vi "UHR-Fleezers Control (host) - 12.0_test_fpga_connection.vi"() -> ()   [LabVIEW 2014] (continued)
                    frame 3 {
                      n2355 = local read "Trap D (MHz)"() -> (w3391:dbl)
                      n2356 = property on="Initial D (MHz)" class="DigNum (strict)"("Val(Sgnl)"=w3391) -> ()  [unwired: 2 in, 2 out]
                      n2357 = local write "Manipulating Trap"(FALSE ("Manipulating Trap")) -> ()
                    }
                  }
                }
              }
            }
          }
        }
      }
      event Mouse Move {
        n2358 = event-data() -> ()  [unwired: 6 out]
      }
    }
    n2359 = local read "Stop All"() -> (w3174:bool)
    n2360 = node-c288() -> ()  [unwired: 2 out]
  }
  n2361 = node-c288(w136) -> ()  [unwired: 1 out]
  n2362 = node-c288(w138) -> ()  [unwired: 1 out]
  n2363 = node-c288(w125) -> ()  [unwired: 1 out]
  n2364 = flat-sequence "Video" {
    tunnel: [w3402] -> w127
    tunnel: w127 -> [w3443]
    frame #0 {
      n2365 = while {
        stop <- w3395 continue-if-true
        n2366 = call "Close Video Capture.vi"() -> ("error code OUT"=w3397:i32)
        n2367 = Equal?(x=w3397, y=0) -> (x = y?=w3395:bool)
      }
      n2368 = local write "Stop All"(FALSE ("Stop All")) -> ()
    }
    frame #1 {
      n2369 = call "DMR_Init.vi"() -> ()  [unwired: 3 out]
    }
    frame #2 {
      # "Setting the destination format to Mono8 makes sure that the image can be displayed in the intensity plot."
      n2370 = call "DMR_GetDevice.vi"("search string IN"="DE019116701") -> ("device handle OUT"=w3420:i32)  [unwired: 4 in, 2 out]
      n2371 = call "DMR_OpenDevice.vi"("device handle IN"=w3420) -> ("driver handle OUT"=w3403:i32)  [unwired: 4 out]
      n2372 = call "DMR_FindList.vi"("flags IN"=u32 0 ("flags"), "list name IN"="" ("String"), "list type IN"=T38."camera descriptions", "driver handle IN"=w3403) -> ("list handle OUT"=w3406:i32)  [unwired: 2 out]
      n2373 = call "DMR_FindList.vi"("flags IN"=u32 0 ("flags"), "list name IN"="Base", "list type IN"=T38."setting", "driver handle IN"=w3403) -> ("list handle OUT"=w3404:i32)  [unwired: 2 out]
      n2374 = call "OBJ_GetHandle.vi"("object name IN"="VideoStandard", "list handle IN"=w3406) -> ("object handle OUT"=w3400:i32)  [unwired: 3 out]
      n2375 = call "OBJ_GetHandle.vi"("object name IN"="PixelFormat", "list handle IN"=w3404) -> ("object handle OUT"=w3414:i32)  [unwired: 3 out]
      n2376 = call "OBJ_SetS.vi"("value index IN"=0, "value IN"="NTSC M", "object handle IN"=w3400) -> ()  [unwired: 2 out]
      n2377 = call "OBJ_SetS.vi"("value index IN"=0, "value IN"="Mono8" ("value"), "object handle IN"=w3414) -> ()  [unwired: 2 out]
      n2378 = call "OBJ_GetHandle.vi"("object name IN"="VideoChannel", "list handle IN"=w3404) -> ("object handle OUT"=w3410:i32)  [unwired: 3 out]
      n2379 = while {
        tunnel: [w3425] -> w3402
        tunnel: w3403 -> [w3422]
        stop <- w3423 continue-if-true
        n2380 = call "DMR_ImageRequestSingle.vi"("request control IN"=0, "driver handle IN"=w3422) -> ("error code OUT"=w3424:i32, "driver handle OUT"=w3425:i32)  [unwired: 2 out]
        n2381 = Equal To 0?(x=w3424) -> (x = 0?=w3423:bool)
      }
      n2382 = call "OBJ_SetI.vi"("value index IN"=0, "value IN"=3 ("Video channel"), "object handle IN"=w3410) -> ()  [unwired: 2 out]
    }
    frame #3 {
      w3431 = T20 0 items=["Grayscale (U8)", "Grayscale (I16)", "Grayscale (SGL)", "Complex (CSG)", "RGB (U32)", "HSL (U32)", "RGB (U64)"] ("Image Type")
      w3439 = T20 0 items=["Grayscale (U8)", "Grayscale (I16)", "Grayscale (SGL)", "Complex (CSG)", "RGB (U32)", "HSL (U32)", "RGB (U64)"] ("Image Type")
      n2383 = for "Create Greyscale map" {
        N: 256 -> [_]
        tunnel: [w3445] -> w3428 mode=indexing
        workers-P: _ -> [_]
        i -> [w3448]
        n2384 = To Unsigned Byte Integer(number=w3448) -> (unsigned 8bit integer=w3444:u8)
        n2385 = Join Numbers(hi=w3444, lo=w3444) -> ((hi.lo)=w3447:u16)
        n2386 = Join Numbers(hi=w3444, lo=w3444) -> ((hi.lo)=w3446:u16)
        n2387 = Join Numbers(hi=w3447, lo=w3446) -> ((hi.lo)=w3445:u32)
      }
      n2388 = call "IMAQ Create"("Image Name"="Scaled video", "Image Type"=w3431) -> ("New Image"=w3430:T2)  [unwired: 2 in, 2 out]
      n2389 = call "IMAQ Create"("Image Name"="Main video", "Image Type"=w3439) -> ("New Image"=w3440:T2)  [unwired: 2 in, 2 out]
      n2390 = node-c288(0 ("Processor")) -> (w3438:T26)  [unwired: 3 out]
      n2391 = Initialize Array(u32 0 ("Window Number (0...15)"), 480 ("dimension size"), 640 ("dimension size")) -> (w3433:u32[][])
      n2392 = timed-loop {
        tunnel: w3443 -> [w3465]
        tunnel: [w3464] -> w3442
        tunnel: w3440 -> [w3463]
        timing: w3438 -> [_]
        timing-out: [_] -> w3437
        tunnel: w3433 -> [w3452]
        tunnel: w3430 -> [w3450]
        tunnel: w3428 -> [w3449]
        stop <- w3451 stop-if-true
        # "This block performs the \nactual image capture."
        n2393 = node-c288() -> ()  [unwired: 2 out]
        n2394 = local read "Stop All"() -> (w3451:bool)
        n2395 = Reciprocal(x="Video Capture Rate (Hz)") -> (1/x=w3455:dbl)
        n2396 = Multiply(x=w3455, y=1000.0) -> (x*y=w3453:dbl)
        n2397 = call "DMR_ImageRequestWaitFor.vi"("queue number IN"=0, "timeout(ms) IN"=500, "driver handle IN"=w3465) -> ("error code OUT"=w3469:i32, "request number OUT"=w3466:i32, "driver handle OUT"=w3467:i32)
        n2398 = feedback #1(T39 refnum ("Avi Refnum")) -> (w3457:T39)
        n2399 = case shown="True" "New Video File" {
          tunnel: [T39 refnum ("Avi Refnum") w3486] -> w3459
          tunnel: [FALSE TRUE] -> w3460
          tunnel: w3457 -> [_ w3482]
          frame False {
          }
          frame True {
            n2400 = call "Create new save file.vi"("Ext"=".avi" ("string"), "Index In"="Video Index") -> ("Path Out"=w3478:path, "Index Out"=w3479:dbl)  [unwired: 1 in]
            "Path Out" <- w3478
            n2401 = Not Equal?(x=w3482, y=T39 refnum ("Avi Refnum")) -> (x != y?=w3483:bool)
            n2402 = Increment(x=w3479) -> (x+1=w3488:dbl)
            n2403 = case shown="True" w3483 {
              tunnel: w3482 -> [_ w3489]
              frame False {
              }
              frame True {
                n2404 = call "IMAQ AVI Close"("Avi Refnum"=w3489) -> ()  [unwired: 1 in, 10 out]
              }
            }
            n2405 = local write "Video Index"(w3488) -> ()
            n2406 = call "IMAQ AVI Create"("Frames Per Second"=u32 30, "AVI Path"=w3478) -> ("Avi Refnum"=w3486:T39)  [unwired: 5 in, 4 out]
          }
        }
        n2407 = Equal To 0?(x=w3469) -> (x = 0?=w3468:bool)
        n2408 = Select(t=w3459, s=w3460, f=w3457) -> (s? t:f=w3458:T39)
        n2409 = feedback-in #1(w3458) -> ()
        n2410 = case shown="True" w3468 {
          tunnel: w3467 -> [w3490 w3517]
          tunnel: w3466 -> [_ w3516]
          tunnel: [w3490 w3513] -> w3464
          tunnel: w3463 -> [_ w3494]
          tunnel: w3452 -> [_ w3501]
          tunnel: w3458 -> [_ w3499]
          tunnel: w3450 -> [_ w3495]
          tunnel: w3449 -> [_ w3496]
          frame False {
          }
          frame True {
            w3507 = u32 0 ("X-offset IN")
            n2411 = call "DMR_GetImageRequestBufferData.vi"("driver handle IN"=w3517, "request number IN"=w3516) -> ("width OUT"=w3506:i32, "height OUT"=w3505:i32, "driver handle OUT"=w3512:i32, "request number OUT"=w3511:i32, "bytes per pixel OUT"=w3508:i32)  [unwired: 13 out]
            n2412 = call "DMR_GetImageRequestBufferImageData.vi"("driver handle IN"=w3512, "request number IN"=w3511, "bytes per pixel IN"=w3508, "X-offset IN"=w3507, "Y-offset IN"=w3507, "height IN"=w3505, "width IN"=w3506) -> ("driver handle OUT"=w3510:u32, "request number OUT"=w3509:u32, "image OUT"=w3502:u32[][])  [unwired: 10 out]
            n2413 = call "DMR_ImageRequestUnlock.vi"("request number IN"=w3509, "driver handle IN"=w3510) -> ("driver handle OUT"=w3515:i32)  [unwired: 1 in, 2 out]
            n2414 = case shown="True" "Averaging" {
              tunnel: w3502 -> [w3558 w3563]
              tunnel: [w3558 w3562] -> w3498
              tunnel: w3501 -> [_ w3560]
              frame False {
              }
              frame True {
                (unwired) 1
                w3568 = 1
                n2415 = feedback #2(w3560) -> (w3559:u32[][])
                n2416 = Add(x=w3563, y=w3559) -> (x+y=w3564:u32[][])
                n2417 = Select(t=w3560, s="Reset Averaging", f=w3564) -> (s? t:f=w3566:u32[][])
                n2418 = feedback-in #2(w3566) -> ()
                n2419 = feedback #3(w3568) -> (w3561:i32)
                n2420 = Divide(x=w3564, y=w3561) -> (x/y=w3565:dbl[][])
                n2421 = Increment(x=w3561) -> (x+1=w3569:i32)
                n2422 = To Unsigned Long Integer(number=w3565) -> (unsigned 32bit integer=w3562:u32[][])
                n2423 = Select(t=w3568, s="Reset Averaging", f=w3569) -> (s? t:f=w3567:i32)
                n2424 = feedback-in #3(w3567) -> ()
              }
            }
            n2425 = call "DMR_ImageRequestSingle.vi"("request control IN"=0, "driver handle IN"=w3515) -> ("driver handle OUT"=w3513:i32)  [unwired: 3 out]
            n2426 = disable-structure shown="Disabled" {
              disable-tunnel: w3498 -> [w3535 _]
              disable-tunnel: w3495 -> [w3534 _]
              frame Disabled {
                n2427 = To Double Precision Float(number=w3535) -> (double precision float=w3533:dbl[][])
                n2428 = In Range and Coerce(upper limit="Intensity Upper", x=w3533, lower limit="Intensity Lower") -> (coerced(x)=w3532:dbl[][])  [unwired: 1 out]
                n2429 = Subtract(x="Intensity Upper", y="Intensity Lower") -> (x-y=w3529:dbl)
                n2430 = Subtract(x=w3532, y="Intensity Lower") -> (x-y=w3530:dbl[][])
                n2431 = Divide(x=w3530, y=w3529) -> (x/y=w3531:dbl[][])
                n2432 = Multiply(x=255.0, y=w3531) -> (x*y=w3527:dbl[][])
                n2433 = To Unsigned Byte Integer(number=w3527) -> (unsigned 8bit integer=w3536:u8[][])
                n2434 = call "IMAQ ArrayToImage"("Image Pixels (U8)"=w3536, "Image"=w3534) -> ("Image Out"=w3523:T2)  [unwired: 4 in, 5 out]
                n2435 = First Call?() -> (First Call?: T/F=w3524:bool)
                n2436 = case shown="True" w3524 {
                  tunnel: w3523 -> [w3537 w3548]
                  frame False {
                    n2437 = flat-sequence {
                      tunnel: w3537 -> [w3543]
                      frame #0 {
                        w3540 = FALSE ("Get/Set Status? (Set)")
                        w3539 = 0 ("Window Number (0...15)")
                        n2438 = call "IMAQ WindSize"("Get/Set Status? (Set)"=w3540, "Window Number"=w3539) -> ("Width & Height out"=→"Window Size":cluster{"Width":i32, "Height":i32})  [unwired: 4 in, 2 out]
                        n2439 = call "IMAQ WindMove"("Window Number (0...15)"=w3539, "Get/Set Status? (Set)"=w3540) -> ("Coordinates (screen)"=→"Window Position":cluster{"X Position":i32, "Y Position":i32})  [unwired: 3 in, 1 out]
                        n2440 = call "IMAQ WindDraw"("Resize to Image Size? (Y)"=FALSE, "Window Number (0...15)"=w3539, "Image"=w3543) -> ()  [unwired: 7 in, 2 out]
                      }
                      frame #1 {
                        n2441 = call "IMAQ WindZoom 2"("Center Point"="Center Point", "Zoom to Fit? (False)"=FALSE, "Zoom Factor"="Zoom Factor") -> ()  [unwired: 5 in, 4 out]
                      }
                    }
                  }
                  frame True {
                    n2442 = flat-sequence {
                      tunnel: w3548 -> [w3551]
                      tunnel: [w3549] -> w3547
                      tunnel: w3547 -> [w3553]
                      frame #0 {
                        w3550 = TRUE ("Resize to Image Size? (Y)")
                        w3549 = 0 ("Window Number (0...15)")
                        n2443 = call "IMAQ WindNonTearing"("Window Number"=w3549, "NonTearing? (True)"=w3550) -> ()  [unwired: 8 in, 2 out]
                        n2444 = call "IMAQ WindDraw"("Resize to Image Size? (Y)"=w3550, "Window Number (0...15)"=w3549, "Image"=w3551) -> ()  [unwired: 7 in, 2 out]
                      }
                      frame #1 {
                        n2445 = call "IMAQ WindSize"("Scrollbars? (N)"=FALSE, "Width & Height"="Initial Window Size", "Window Number"=w3553) -> ()  [unwired: 3 in, 3 out]
                        n2446 = call "IMAQ WindMove"("Window Number (0...15)"=w3553, "Coordinates (screen)"="Initial Window Position") -> ()  [unwired: 3 in, 2 out]
                      }
                    }
                  }
                }
              }
              frame Enabled {
              }
            }
            n2447 = To Unsigned Byte Integer(number=w3498) -> (unsigned 8bit integer=w3497:u8[][])
            n2448 = call "IMAQ ArrayToImage"("Image Pixels (U8)"=w3497, "Image"=w3494) -> ("Image Out"=w3492:T2)  [unwired: 4 in, 5 out]
            n2449 = case shown="True" "Save Video" {
              tunnel: w3499 -> [_ w3557]
              tunnel: w3492 -> [_ w3556]
              frame False {
              }
              frame True {
                n2450 = call "IMAQ AVI Write Frame"("Image"=w3556, "Avi Refnum"=w3557) -> ()  [unwired: 2 in, 8 out]
              }
            }
            n2451 = case shown="True" "Save Image" {
              tunnel: w3497 -> [_ w3572]
              tunnel: w3496 -> [_ w3571]
              frame False {
              }
              frame True {
                n2452 = call <vilib>:"Flatten Pixmap.vi"("colors"=w3571, "8-bit pixmap"=w3572) -> ("image data"=w3578:T40)  [unwired: 4 in, 5 out]
                n2453 = call "Create new save file.vi"("Insert"="video_frame_" ("string"), "Ext"=".bmp" ("string"), "Index In"="Image Index") -> ("Path Out"=w3574:path, "Index Out"=w3579:dbl)
                n2454 = Increment(x=w3579) -> (x+1=w3573:dbl)
                n2455 = local write "Image Index"(w3573) -> ()
                n2456 = call <vilib>:"Write BMP File.vi"("image data"=w3578, "path to BMP file"=w3574) -> ()  [unwired: 1 in, 9 out]
              }
            }
            n2457 = case shown="True" "Target" {
              tunnel: w3492 -> [w3518 w3522]
              tunnel: [w3518 w3520] -> w3491
              frame False {
              }
              frame True {
                n2458 = local read "Target coordinates"() -> (w3519:cluster{"X1":dbl, "Y1":dbl, "X2":dbl, "Y2":dbl})
                n2459 = call "IMAQ Overlay Oval"("Color"=u32 16711680, "Bounding Rectangle"=w3519, "Image"=w3522) -> ("Image Out"=w3520:T2)  [unwired: 7 in, 1 out]
              }
            }
            "Primary Video Display" <- w3491
          }
        }
        n2460 = node-c288(w3453) -> ()  [unwired: 1 out]
      }
      n2461 = node-c288(w3437) -> ()  [unwired: 1 out]
      n2462 = call "DMR_CloseDevice2.vi"("driver handle IN"=w3442) -> ()  [unwired: 1 in, 4 out]
    }
    frame #4 {
      n2463 = call "DMR_Close.vi"() -> ()  [unwired: 1 out]
    }
  }
  n2464 = local write "Offset (nm)"(0.0 ("Offset (nm)")) -> ()
  n2465 = local write "Bead Mean (nm)"(0.0 ("Bead Mean (nm)")) -> ()
  n2466 = local write "Total Volume\nFlowed P1 (uL)"(w45) -> ()
  n2467 = local write "Total Volume\nFlowed Samp (uL)"(w45) -> ()
  n2468 = local write "Total Volume\nFlowed P3 (uL)"(w45) -> ()
  n2469 = node-c288(i64 1 ("Period"), 1 ("Processor")) -> (w217:T26)  [unwired: 2 out]
  n2470 = timed-loop "Acquire Data" {
    tunnel: w51 -> [w3886]
    tunnel: w98 -> [w3885]
    tunnel: [w3915] -> w309
    tunnel: [w3910] -> w307
    timing: w217 -> [_]
    timing-out: [_] -> w216
    tunnel: w116 -> [w3742]
    stop <- "Stop All" stop-if-true
    w3666 = "Initialize"
    w3732 = "NI_ChannelName" ("name")
    # "I think that the conversion\nfrom 'wiggle amp' to nm\nis 0.277 nm/input. So, 1000\nfor an input is 277 nm."
    n2471 = node-c288() -> ()  [unwired: 2 out]
    n2472 = First Call?() -> (First Call?: T/F=w3701:bool)
    n2473 = Or(x="Reset", y=w3701) -> (x .or. y?=w3702:bool)
    n2474 = local read "Flushing P1"() -> (w3621:bool)
    n2475 = case "Reset data stream" shown="True" w3702 {
      tunnel: w3886 -> [w4951 w4959]
      tunnel: w3885 -> [w4950 w4958]
      tunnel: [w4951 w4953] -> w3614
      tunnel: [w4950 w4952] -> w3881
      frame False {
      }
      frame True {
        w4956 = TRUE ("AI to FIFO")
        n2476 = local write "Overflow (data lost)"(FALSE ("Overflow (data lost)")) -> ()
        n2477 = call "reset FPGA DMA.vi"("error in"=w4958, "FPGA VI Reference In"=w4959) -> ("error out"=w4954:errorcluster, "FPGA VI Reference Out"=w4955:T22)
        n2478 = xnode "Read/Write Control"("FPGA VI Reference In"=w4955, "error in"=w4954, "AI to FIFO"=w4956, "APD to FIFO"=w4956) -> ("FPGA VI Reference Out"=w4953:T22, "error out"=w4952:errorcluster)
      }
    }
    n2479 = case shown="True" w3621 {
      frame False {
      }
      frame True {
        n2480 = local read "Flush rate (uL/m) P1"() -> (w3986:dbl)
        n2481 = local read "HP1 Flush Time (s)"() -> (w3992:dbl)
        n2482 = local read "DMA Update Period (s)"() -> (w3979:dbl)
        n2483 = Divide(x=w3986, y=60.0) -> (x/y=w3978:dbl)
        n2484 = feedback #4(0.0) -> (w3981:dbl)
        n2485 = Divide(x=w3992, y=w3979) -> (x/y=w3984:dbl)
        n2486 = feedback #5(0) -> (w3990:i32)
        n2487 = Increment(x=w3990) -> (x+1=w3983:i32)
        n2488 = Multiply(x=w3979, y=w3978) -> (x*y=w3977:dbl)
        n2489 = Greater?(x=w3983, y=w3984) -> (0:w3989:bool)
        n2490 = Compound Arithmetic op=MULTIPLY(w3979, w3983, w3978) -> (→"P1 Flush Volume (uL)":dbl)
        n2491 = Divide(x=w3983, y=w3984) -> (x/y=→"P1 Flushing Bar":dbl)
        n2492 = Add(x=w3977, y=w3981) -> (x+y=w3980:dbl)
        "Total Volume\nFlowed P1 (uL)" <- w3980
        n2493 = feedback-in #4(w3980) -> ()
        n2494 = case shown="True" w3989 {
          tunnel: w3983 -> [w3993 _]
          tunnel: [w3993 0] -> w3988
          frame False {
          }
          frame True {
            w3994 = FALSE ("Flushing P1")
            n2495 = local write "Inject Pump 1"(w3994) -> ()
            n2496 = local write "Flushing P1"(w3994) -> ()
            n2497 = property on="Clear Volume P1" class="Bool (strict)"("Val(Sgnl)"=TRUE ("Value (Signaling)")) -> ()  [unwired: 2 in, 2 out]
          }
        }
        n2498 = feedback-in #5(w3988) -> ()
      }
    }
    n2499 = Or(x="Start AOD Scan", y="Trap Raster Scan") -> (x .or. y?=w3840:bool)
    n2500 = case "Start AOM raster scan" shown="True" w3840 {
      tunnel: w3614 -> [w4801 w4811]
      tunnel: w3881 -> [w4800 w4810]
      tunnel: [w4801 w4804] -> w3606
      tunnel: [w4800 w4803] -> w3880
      frame False {
      }
      frame True {
        n2501 = case shown="True" "Restart DMA? (AOD)" {
          tunnel: [w4849 w4851] -> w4805
          tunnel: [w4848 w4850] -> w4806
          tunnel: w4811 -> [w4849 w4853]
          tunnel: w4810 -> [w4848 w4852]
          frame False {
          }
          frame True {
            n2502 = local write "Overflow (data lost)"(FALSE ("Overflow (data lost)")) -> ()
            n2503 = call "reset FPGA DMA.vi"("error in"=w4852, "FPGA VI Reference In"=w4853) -> ("error out"=w4850:errorcluster, "FPGA VI Reference Out"=w4851:T22)
          }
        }
        n2504 = local write "Trap Raster Scan"(FALSE ("Trap Raster Scan")) -> ()
        n2505 = case shown="False" "Move MCL Also?" {
          tunnel: w4806 -> [w4815 w4843]
          tunnel: w4805 -> [w4816 w4844]
          tunnel: [w4814 w4847] -> w4804
          tunnel: [w4813 w4846] -> w4803
          frame False {
            w4812 = TRUE ("AI to FIFO")
            n2506 = xnode "Read/Write Control"("FPGA VI Reference In"=w4816, "error in"=w4815, "AI to FIFO"=w4812, "APD to FIFO"=w4812, "Start scan"=w4812) -> ("FPGA VI Reference Out"=w4814:T22, "error out"=w4813:errorcluster)
          }
          frame True {
            w4840 = FALSE ("1D or 2D Scan?")
            w4845 = TRUE ("AI to FIFO")
            # "Count for MCL loop"
            # "N total cycles"
            # "N steps"
            # "V_int"
            n2507 = local read "Scan Range (nm)"() -> (w4822:dbl)
            n2508 = local read "Number of F/B Scans (AOD)"() -> (w4839:u16)
            n2509 = Sign(1:w4822) -> (0:w4821:dbl)
            n2510 = Compound Arithmetic op=MULTIPLY(w4822, "MCL Step Position Ratio", "MCL/AOM Scale Tweak") -> (w4826:dbl)
            n2511 = Negate(x=w4821) -> (-x=w4818:dbl)
            n2512 = Multiply(x=w4818, y="MCL Step Increment (V_int)") -> (x*y=w4820:dbl)
            n2513 = Divide(x=w4826, y="MCL X Cal (nm/V)") -> (x/y=w4832:dbl)
            n2514 = Multiply(x=32767.0 ("y"), y=w4832) -> (x*y=w4838:dbl)
            n2515 = local read "Total Counts (ticks)"() -> (w4823:u32)
            n2516 = local read "Cycles/step (AOD)"() -> (w4834:u64)
            n2517 = local read "Scan steps (AOD)"() -> (w4835:u64)
            n2518 = Divide(x=w4838, y=10.0) -> (x/y=w4831:dbl)
            n2519 = Divide(x=w4831, y="MCL Step Increment (V_int)") -> (x/y=w4829:dbl)
            n2520 = Absolute Value(x=w4829) -> (abs(x)=w4817:dbl)
            n2521 = Compound Arithmetic op=MULTIPLY(w4835, w4834, w4823) -> (w4830:u64)
            n2522 = local write "wait to reset values"(w4845) -> ()
            n2523 = local write "MCL Scanning"(w4845) -> ()
            n2524 = Divide(x=w4830, y=w4817) -> (x/y=w4827:dbl)
            "MCL Count" <- w4827
            n2525 = xnode "Read/Write Control"("FPGA VI Reference In"=w4844, "error in"=w4843, "Scan steps (MCL)"=w4817, "Number of scans (MCL)"=w4839, "Cycles per step (MCL)"=u64 1, "Scan freq.  increment (MCL)"=w4820, "1D or 2D Scan?"=w4840, "MCL Scan Axis"=w4840, "Cont. Scan (MCL)"=w4840, "MCL count"=w4827) -> ("FPGA VI Reference Out"=w4842:T22, "error out"=w4841:errorcluster)
            n2526 = xnode "Read/Write Control"("FPGA VI Reference In"=w4842, "error in"=w4841, "AI to FIFO"=w4845, "APD to FIFO"=w4845, "Start scan"=w4845, "Start scan (MCL)"=w4845) -> ("FPGA VI Reference Out"=w4847:T22, "error out"=w4846:errorcluster)
          }
        }
        "Raster Scanning..." <- TRUE ("Scanning...")
      }
    }
    n2527 = local read "Flushing P3"() -> (w3622:bool)
    n2528 = case "Keep track of when Harvard Pump 3 is done flushing" shown="True" w3622 {
      frame False {
      }
      frame True {
        n2529 = local read "Flush rate (uL/m) P3"() -> (w4005:dbl)
        n2530 = local read "DMA Update Period (s)"() -> (w3999:dbl)
        n2531 = local read "HP3 Flush Time (s)"() -> (w4013:dbl)
        n2532 = Divide(x=w4005, y=60.0) -> (x/y=w4000:dbl)
        n2533 = feedback #6(0) -> (w4011:i32)
        n2534 = Increment(x=w4011) -> (x+1=w4006:i32)
        n2535 = Divide(x=w4013, y=w3999) -> (x/y=w4007:dbl)
        n2536 = Multiply(x=w3999, y=w4000) -> (x*y=w3998:dbl)
        n2537 = Greater?(x=w4006, y=w4007) -> (0:w4010:bool)
        n2538 = feedback #7(0.0) -> (w4001:dbl)
        n2539 = Compound Arithmetic op=MULTIPLY(w3999, w4006, w4000) -> (→"P3 Flush Volume (uL)":dbl)
        n2540 = case shown="True" w4010 {
          tunnel: w4006 -> [w4014 _]
          tunnel: [w4014 0] -> w4009
          frame False {
          }
          frame True {
            w4015 = FALSE ("Flushing P3")
            n2541 = local write "Inject Pump 3"(w4015) -> ()
            n2542 = local write "Flushing P3"(w4015) -> ()
            n2543 = property on="Clear Volume P3" class="Bool (strict)"("Val(Sgnl)"=TRUE ("Value (Signaling)")) -> ()  [unwired: 2 in, 2 out]
          }
        }
        n2544 = feedback-in #6(w4009) -> ()
        n2545 = Divide(x=w4006, y=w4007) -> (x/y=→"P3 Flushing Bar":dbl)
        n2546 = Add(x=w3998, y=w4001) -> (x+y=w4002:dbl)
        "Total Volume\nFlowed P3 (uL)" <- w4002
        n2547 = feedback-in #7(w4002) -> ()
      }
    }
    n2548 = And(x="Save scans", y=w3840) -> (x .and. y?=w3879:bool)
    n2549 = local read "Flushing samp"() -> (w3615:bool)
    n2550 = case shown="True" w3615 {
      frame False {
      }
      frame True {
        n2551 = local read "DMA Update Period (s)"() -> (w3958:dbl)
        n2552 = local read "Flush rate (mL/m)"() -> (w3970:dbl)
        n2553 = local read "Samp Flush Time (s)"() -> (w3971:dbl)
        n2554 = Divide(x=w3970, y=60.0) -> (x/y=w3957:dbl)
        n2555 = feedback #8(0) -> (w3963:i32)
        n2556 = Increment(x=w3963) -> (x+1=w3962:i32)
        n2557 = Divide(x=w3971, y=w3958) -> (x/y=w3967:dbl)
        n2558 = Multiply(x=w3958, y=w3957) -> (x*y=w3956:dbl)
        n2559 = Greater?(x=w3962, y=w3967) -> (0:w3966:bool)
        n2560 = feedback #9(0.0) -> (w3959:dbl)
        n2561 = Compound Arithmetic op=MULTIPLY(w3958, w3962, w3957) -> (→"Samp Volume (uL)":dbl)
        n2562 = Divide(x=w3962, y=w3967) -> (x/y=→"Samp flush bar":dbl)
        n2563 = case shown="True" w3966 {
          tunnel: [w3972 0] -> w3965
          tunnel: w3962 -> [w3972 _]
          frame False {
          }
          frame True {
            w3975 = FALSE ("Flushing samp")
            n2564 = local write "Sample Channel\nFlow"(w3975) -> ()
            n2565 = local write "Flushing samp"(w3975) -> ()
            n2566 = property on="Clear Volume" class="Bool (strict)"("Val(Sgnl)"=TRUE) -> ()  [unwired: 2 in, 2 out]
          }
        }
        n2567 = feedback-in #8(w3965) -> ()
        n2568 = Add(x=w3956, y=w3959) -> (x+y=w3960:dbl)
        "Total Volume\nFlowed Samp (uL)" <- w3960
        n2569 = feedback-in #9(w3960) -> ()
      }
    }
    n2570 = Compound Arithmetic op=OR("Start MCL Scan", "Confocal\nImage", "Confocal\nLinescan") -> (w3838:bool)
    n2571 = And(x="Save Data (MCL)", y=w3838) -> (x .and. y?=w3878:bool)
    n2572 = case "Start MCL raster scan" shown="True" w3838 {
      tunnel: w3606 -> [w4420 w4436]
      tunnel: w3880 -> [w4419 w4435]
      tunnel: [w4420 w4431] -> w3613
      tunnel: [w4419 w4430] -> w3611
      tunnel: [FALSE w4429] -> w3864
      tunnel: "Start MCL Scan" -> [_ w4424]
      tunnel: "Confocal\nImage" -> [_ w4423]
      tunnel: "Confocal\nLinescan" -> [_ _]
      frame False {
      }
      frame True {
        w4429 = TRUE
        n2573 = case shown="True" "Restart DMA? (MCL)" {
          tunnel: [w4481 w4483] -> w4434
          tunnel: [w4480 w4482] -> w4433
          tunnel: w4436 -> [w4481 w4486]
          tunnel: w4435 -> [w4480 w4485]
          frame False {
          }
          frame True {
            n2574 = call "reset FPGA DMA.vi"("error in"=w4485, "FPGA VI Reference In"=w4486) -> ("error out"=w4482:errorcluster, "FPGA VI Reference Out"=w4483:T22)
            n2575 = local write "Overflow (data lost)"(FALSE ("Overflow (data lost)")) -> ()
          }
        }
        n2576 = case shown="False" w4424 {
          selector: w4424 -> [_ w4440]
          tunnel: w4423 -> [w4439 _]
          tunnel: [w4439 w4440] -> w4422
          frame False {
            n2577 = property on="2D or 1D Scan" class="Bool (strict)"("Val(Sgnl)"=w4439) -> ()  [unwired: 2 in, 2 out]
            n2578 = property on="Confocal\nImage" class="Bool (strict)"("Value"=FALSE ("Start Confocal Map")) -> ()  [unwired: 2 in, 2 out]
          }
          frame True {
          }
        }
        n2579 = local write "MCL Scanning"(w4429) -> ()
        n2580 = local read "AO1"() -> (w4426:dbl)
        n2581 = local read "AO2"() -> (w4425:dbl)
        n2582 = case shown="True" "Center Scan" {
          tunnel: w4434 -> [w4447 w4479]
          tunnel: w4433 -> [w4446 w4478]
          tunnel: [w4445 w4477] -> w4431
          tunnel: [w4444 w4476] -> w4430
          tunnel: [w4442 w4463] -> w4428
          tunnel: [w4441 w4462] -> w4427
          tunnel: w4426 -> [w4442 w4468]
          tunnel: w4425 -> [w4441 w4471]
          tunnel: w4422 -> [_ _]
          frame False {
            w4443 = TRUE ("AI to FIFO")
            n2583 = xnode "Read/Write Control"("FPGA VI Reference In"=w4447, "error in"=w4446, "AI to FIFO"=w4443, "APD to FIFO"=w4443, "Start scan (MCL)"=w4443) -> ("FPGA VI Reference Out"=w4445:T22, "error out"=w4444:errorcluster)
          }
          frame True {
            w4475 = TRUE ("AI to FIFO")
            n2584 = local read "Scan steps (MCL)"() -> (w4454:u64)
            n2585 = local read "Scan lines (y)"() -> (w4450:u64)
            n2586 = local read "Fast Scan Dir"() -> (w4461:bool)
            n2587 = local read "Actual MCL Inc (V)"() -> (w4451:dbl)
            n2588 = Decrement(x=w4450) -> (x-1=w4449:u64)
            n2589 = Decrement(x=w4454) -> (x-1=w4453:u64)
            n2590 = Multiply(x=w4451, y=w4449) -> (x*y=w4448:dbl)
            n2591 = Divide(x=w4448, y=2.0) -> (x/y=w4458:dbl)
            n2592 = Multiply(x=w4451, y=w4453) -> (x*y=w4452:dbl)
            n2593 = Divide(x=w4452, y=2.0) -> (x/y=w4457:dbl)
            n2594 = Select(t=w4457, s=w4461, f=w4458) -> (s? t:f=w4456:dbl)
            n2595 = Select(t=w4458, s=w4461, f=w4457) -> (s? t:f=w4460:dbl)
            n2596 = Subtract(x=w4468, y=w4460) -> (x-y=w4459:dbl)
            n2597 = Subtract(x=w4471, y=w4456) -> (x-y=w4455:dbl)
            n2598 = local read "2D or 1D Scan"() -> (w4473:bool)
            n2599 = Not(x=w4461) -> (.not. x?=w4467:bool)
            n2600 = Not(x=w4473) -> (.not. x?=w4469:bool)
            n2601 = And(x=w4461, y=w4469) -> (x .and. y?=w4470:bool)
            n2602 = And(x=w4469, y=w4467) -> (x .and. y?=w4472:bool)
            n2603 = Select(t=w4471, s=w4472, f=w4455) -> (s? t:f=w4462:dbl)
            n2604 = Select(t=w4468, s=w4470, f=w4459) -> (s? t:f=w4463:dbl)
            n2605 = call "Volt to I16.vi"("Voltage In"=w4463) -> ("I16 Voltage Out"=w4466:i16)
            n2606 = call "Volt to I16.vi"("Voltage In"=w4462) -> ("I16 Voltage Out"=w4465:i16)
            n2607 = xnode "Read/Write Control"("FPGA VI Reference In"=w4479, "error in"=w4478, "AI to FIFO"=w4475, "APD to FIFO"=w4475, "Start scan (MCL)"=w4475, "AO1"=w4466, "AO2"=w4465) -> ("FPGA VI Reference Out"=w4477:T22, "error out"=w4476:errorcluster)
          }
        }
        "Initial Y" <- w4428
        "Initial X" <- w4427
        n2608 = local write "Tab Control 6"(T3."Imaging" ("Tab Control 6")) -> ()
        "wait to reset values" <- w4429
      }
    }
    n2609 = case shown="True" "Wiggle" {
      selector: "Wiggle" -> [w3929 _]
      tunnel: w3613 -> [w3931 w3944]
      tunnel: [w3928 w3947] -> w3612
      tunnel: w3611 -> [w3930 w3942]
      tunnel: [w3927 w3946] -> w3610
      frame False {
        n2610 = xnode "Read/Write Control"("FPGA VI Reference In"=w3931, "error in"=w3930, "Wiggle trap 1"=w3929) -> ("FPGA VI Reference Out"=w3928:T22, "error out"=w3927:errorcluster)
      }
      frame True {
        w3936 = FALSE ("Abort wiggle")
        w3940 = TRUE
        n2611 = local read "Restart DMA? (AOD)"() -> (w3945:bool)
        n2612 = case shown="True" w3945 {
          tunnel: w3944 -> [w3949 w3954]
          tunnel: [w3949 w3953] -> w3943
          tunnel: w3942 -> [w3948 w3952]
          tunnel: [w3948 w3951] -> w3941
          frame False {
          }
          frame True {
            n2613 = local write "Overflow (data lost)"(FALSE) -> ()
            n2614 = call "reset FPGA DMA.vi"("error in"=w3952, "FPGA VI Reference In"=w3954) -> ("error out"=w3951:errorcluster, "FPGA VI Reference Out"=w3953:T22)
          }
        }
        n2615 = local write "Wiggle"(FALSE) -> ()
        n2616 = xnode "Read/Write Control"("FPGA VI Reference In"=w3943, "error in"=w3941, "AI to FIFO"=w3940, "APD to FIFO"=w3940, "Wiggle trap 1"="Wiggle T1", "Wiggle freq 1 (Hz)"="Wiggle freq 1 (Hz)", "Wiggle amp 1"="Wiggle amp 1 (units?)", "Abort wiggle 1"=w3936, "Wiggle trap 2"="Wiggle T2", "Abort wiggle 2"=w3936, "Wiggle freq 2 (Hz)"="Wig Freq 2 (Hz)", "Wiggle amp 2"="Wig amp 2") -> ("FPGA VI Reference Out"=w3947:T22, "error out"=w3946:errorcluster)
      }
    }
    n2617 = local read "Trap Pos Elements/DMA read"() -> (w3596:u32)
    n2618 = local read "Trap AI Elements/DMA read"() -> (w3590:u32)
    n2619 = local read "APD Elements/DMA read"() -> (w3598:u32)
    n2620 = xnode "Get APD Data"("FPGA VI Reference In"=w3612, "error in"=w3610, "Number of Elements"=w3598, "Timeout (ms)"=-1) -> ("Data"=w3774:u32[], "Elements Remaining"=→"APD FIFO Elements Remaining":u32)  [unwired: 2 out]
    n2621 = xnode "Invoke Method"("FPGA VI Reference In"=w3612, "error in"=w3610, "Number of Elements"=w3596, "Timeout (ms)"=-1) -> ("Data"=w3705:u16[], "Elements Remaining"=→"Trap Pos FIFO El Remaining":u32)  [unwired: 2 out]
    n2622 = xnode "Get Trap Data"("FPGA VI Reference In"=w3612, "error in"=w3610, "Number of Elements"=w3590, "Timeout (ms)"=-1 ("Timeout")) -> ("FPGA VI Reference Out"=w3643:T22, "error out"=w3642:errorcluster, "Data"=w3706:i16[], "Elements Remaining"=w3589:u32)
    "FIFO El. Rem." <- w3589
    n2623 = local read "Trap AI FIFO Depth"() -> (w3924:u32)
    n2624 = Subtract(x=w3924, y=w3590) -> (x-y=w3923:u32)
    n2625 = Decimate 1D Array(w3705) -> (w3594:u16[], w3592:u16[], w3593:u16[])
    n2626 = Divide(x=w3589, y=w3923) -> (x/y=w3922:dbl)
    "Buffer Status" <- w3922
    n2627 = To Unsigned Long Integer(number=w3594) -> (unsigned 32bit integer=w3704:u32[])
    n2628 = Join Numbers(hi=w3592, lo=w3593) -> ((hi.lo)=w3703:u32[])
    n2629 = Equal?(x=w3922, y=1.0) -> (x = y?=w3920:bool)
    n2630 = Join Numbers(hi=w3704, lo=w3703) -> ((hi.lo)=w3697:u64[])
    n2631 = call "IR AOM word to freq - vec.vi"("Frequency Word In (double vec)"=w3697) -> ("Frequency Out"=w3740:dbl[])
    n2632 = case "Alert buffer overflow" shown="True" w3920 {
      frame False {
      }
      frame True {
        n2633 = call <vilib>:"Beep.vi"() -> ()  [unwired: 3 in, 9 out]
        "Overflow (data lost)" <- TRUE ("Overflow (data lost)")
      }
    }
    n2634 = Decimate 1D Array(w3740) -> (w3739:dbl[], w3738:dbl[])
    n2635 = Build Array(w3739, w3738) -> (w3737:dbl[][])
    n2636 = local read "Trap Sets"() -> (w3804:u32)
    n2637 = case "Deinterlace trap data, average down PSD" shown="2" w3804 {
      tunnel: w3706 -> [w4512 w4581]
      tunnel: [w4515 w4578] -> w3797
      tunnel: [w4512 w4580] -> w3700
      tunnel: "Detector Type" -> [w4517 w4576]
      tunnel: [w4516 w4579] -> w3796
      tunnel: [w4514 w4577] -> w3897
      frame 1, Default {
        n2638 = Divide(x=w4512, y=3276.7) -> (x/y=w4513:dbl[])
        n2639 = Decimate 1D Array(w4513) -> (w4526:dbl[], w4525:dbl[], w4524:dbl[], w4523:dbl[], w4522:dbl[], w4521:dbl[], w4520:dbl[], w4519:dbl[])
        n2640 = case shown="\"IR-QPD + PSD + FB-QPD position\"" w4517 {
          tunnel: w4526 -> [w4550 w4575]
          tunnel: w4525 -> [w4549 w4574]
          tunnel: w4524 -> [w4534 w4552]
          tunnel: w4523 -> [w4535 w4562]
          tunnel: w4522 -> [w4548 w4573]
          tunnel: w4521 -> [w4547 w4572]
          tunnel: w4520 -> [w4531 w4553]
          tunnel: w4519 -> [w4530 w4551]
          tunnel: [w4529 w4559] -> w4516
          tunnel: [w4528 w4558] -> w4515
          tunnel: [w4527 w4557] -> w4514
          frame "IR-QPD + PSD + FB-QPD", Default {
            w4527 = 0  # Channel pattern
            n2641 = Divide(x=w4550, y=w4535) -> (x/y=w4537:dbl[])
            n2642 = Divide(x=w4549, y=w4535) -> (x/y=w4536:dbl[])
            n2643 = Divide(x=w4548, y=w4531) -> (x/y=w4533:dbl[])
            n2644 = Divide(x=w4547, y=w4530) -> (x/y=w4532:dbl[])
            n2645 = Build Array(w4537, w4536, w4535, w4534, w4533, w4532, w4531, w4530) -> (w4528:dbl[][])
            n2646 = Bundle("T1 Y", "T1 X", "T1 Sum", "FB Sum", "PSD Y", "PSD X", "PSD Y Sum", "PSD X Sum") -> (w4546:T47)  [unwired: 1 out]
            n2647 = Cluster To Array(cluster=w4546) -> (array=w4529:string[])
          }
          frame "IR-QPD + PSD + FB-QPD position" {
            w4557 = 3  # Channel pattern
            n2648 = Negate(x=w4553) -> (-x=w4554:dbl[])
            n2649 = Divide(x=w4575, y=w4562) -> (x/y=w4564:dbl[])
            n2650 = Divide(x=w4574, y=w4562) -> (x/y=w4563:dbl[])
            n2651 = Divide(x=w4573, y=w4553) -> (x/y=w4561:dbl[])
            n2652 = Divide(x=w4572, y=w4554) -> (x/y=w4560:dbl[])
            n2653 = Build Array(w4564, w4563, w4562, w4551, w4552, w4561, w4560, w4553) -> (w4558:dbl[][])
            n2654 = Bundle("T1 Y", "T1 X", "T1 Sum", "FB X", "FB Sum", "PSD Y", "PSD X", "PSD Y Sum") -> (w4571:T47)  [unwired: 1 out]
            n2655 = Cluster To Array(cluster=w4571) -> (array=w4559:string[])
          }
        }
      }
      frame 2 {
        n2656 = case shown="\"IR-QPD + PSD + FB-QPD XY positions\"" w4576 {
          tunnel: w4581 -> [w4643 w4710 w4779]
          tunnel: [w4594 w4706 w4724] -> w4580
          tunnel: [w4619 w4698 w4765] -> w4579
          tunnel: [w4618 w4665 w4736] -> w4578
          tunnel: [w4614 w4696 w4763] -> w4577
          frame "IR-QPD + PSD + FB-QPD", Default {
            w4614 = 1  # Channel pattern
            # "time average x2 the 4th signal and the 4 psd signals (detection laser)"
            # "deinterlace 3 signals from qpd"
            n2657 = Decimate 1D Array(w4643) -> (w4642:i16[], w4641:i16[], w4617:i16[], w4640:i16[], w4593:i16[], w4592:i16[], w4591:i16[], w4590:i16[])
            n2658 = Decimate 1D Array(w4617) -> (w4583:i16[], w4582:i16[])
            n2659 = Decimate 1D Array(w4642) -> (w4589:i16[], w4588:i16[])
            n2660 = Decimate 1D Array(w4641) -> (w4587:i16[], w4585:i16[])
            n2661 = Decimate 1D Array(w4640) -> (w4586:i16[], w4584:i16[])
            n2662 = call "downsample 1D array - double.vi"("Ave N"=2.0, "Array In"=w4593) -> ("Array Out"=w4635:dbl[])  [unwired: 1 out]
            n2663 = call "downsample 1D array - double.vi"("Ave N"=2.0, "Array In"=w4592) -> ("Array Out"=w4620:dbl[])  [unwired: 1 out]
            n2664 = call "downsample 1D array - double.vi"("Ave N"=2.0, "Array In"=w4591) -> ("Array Out"=w4634:dbl[])  [unwired: 1 out]
            n2665 = call "downsample 1D array - double.vi"("Ave N"=2.0, "Array In"=w4590) -> ("Array Out"=w4633:dbl[])  [unwired: 1 out]
            n2666 = Interleave 1D Arrays(w4589, w4587, w4586, w4588, w4585, w4584, w4583, w4582, w4635, w4620, w4634, w4633) -> (w4632:dbl[])
            n2667 = Divide(x=w4632, y=3276.7) -> (x/y=w4631:dbl[])
            n2668 = Decimate 1D Array(w4631) -> (w4630:dbl[], w4629:dbl[], w4628:dbl[], w4627:dbl[], w4626:dbl[], w4625:dbl[], w4616:dbl[], w4615:dbl[], w4624:dbl[], w4623:dbl[], w4622:dbl[], w4621:dbl[])
            n2669 = Divide(x=w4630, y=w4628) -> (x/y=w4601:dbl[])
            n2670 = Divide(x=w4629, y=w4628) -> (x/y=w4600:dbl[])
            n2671 = Divide(x=w4627, y=w4625) -> (x/y=w4599:dbl[])
            n2672 = Divide(x=w4626, y=w4625) -> (x/y=w4598:dbl[])
            n2673 = Divide(x=w4624, y=w4622) -> (x/y=w4597:dbl[])
            n2674 = Divide(x=w4623, y=w4621) -> (x/y=w4596:dbl[])
            n2675 = Build Array(w4601, w4600, w4628, w4599, w4598, w4625, w4616, w4615, w4597, w4596, w4622, w4621) -> (w4618:dbl[][])
            n2676 = Bundle("T1 Y", "T1 X", "T1 Sum", "T2 Y", "T2 X", "T2 Sum", "T1 FB Sum", "T2 FB Sum", "PSD Y", "PSD X", "PSD Y Sum", "PSD X Sum") -> (w4602:T48)  [unwired: 1 out]
            n2677 = To Word Integer(number=w4632) -> (16bit integer=w4594:i16[])
            n2678 = Cluster To Array(cluster=w4602) -> (array=w4619:string[])
          }
          frame "IR-QPD + PSD + FB-QPD X position" {
            w4696 = 2  # Channel pattern
            # "time average x2 the 3 psd signals (detection laser)"
            # "deinterlace 3 signals from qpds"
            n2679 = Decimate 1D Array(w4710) -> (w4709:i16[], w4708:i16[], w4697:i16[], w4707:i16[], w4657:i16[], w4656:i16[], w4655:i16[], w4684:i16[])
            n2680 = Decimate 1D Array(w4697) -> (w4647:i16[], w4645:i16[])
            n2681 = Decimate 1D Array(w4709) -> (w4654:i16[], w4651:i16[])
            n2682 = Decimate 1D Array(w4708) -> (w4653:i16[], w4650:i16[])
            n2683 = Decimate 1D Array(w4707) -> (w4652:i16[], w4649:i16[])
            n2684 = Decimate 1D Array(w4684) -> (w4648:i16[], w4646:i16[])
            n2685 = call "downsample 1D array - I16.vi"("Ave N"=2.0, "Array In"=w4657) -> ("Array Out"=w4662:i16[])  [unwired: 1 in]
            n2686 = call "downsample 1D array - I16.vi"("Ave N"=2.0, "Array In"=w4655) -> ("Array Out"=w4658:i16[])  [unwired: 1 in]
            n2687 = call "downsample 1D array - I16.vi"("Ave N"=2.0, "Array In"=w4656) -> ("Array Out"=w4660:i16[])  [unwired: 1 in]
            n2688 = Interleave 1D Arrays(w4654, w4653, w4652, w4651, w4650, w4649, w4648, w4647, w4646, w4645, w4662, w4660, w4658) -> (w4706:i16[])
            n2689 = Divide(x=w4706, y=3276.7) -> (x/y=w4705:dbl[])
            n2690 = Decimate 1D Array(w4705) -> (w4704:dbl[], w4703:dbl[], w4702:dbl[], w4701:dbl[], w4700:dbl[], w4699:dbl[], w4676:dbl[], w4674:dbl[], w4673:dbl[], w4671:dbl[], w4670:dbl[], w4669:dbl[], w4666:dbl[])
            n2691 = Negate(x=w4666) -> (-x=w4664:dbl[])
            n2692 = Divide(x=w4670, y=w4666) -> (x/y=w4668:dbl[])
            n2693 = Divide(x=w4669, y=w4664) -> (x/y=w4667:dbl[])
            n2694 = Divide(x=w4704, y=w4702) -> (x/y=w4688:dbl[])
            n2695 = Divide(x=w4703, y=w4702) -> (x/y=w4687:dbl[])
            n2696 = Divide(x=w4701, y=w4699) -> (x/y=w4686:dbl[])
            n2697 = Divide(x=w4700, y=w4699) -> (x/y=w4685:dbl[])
            n2698 = Divide(x=w4676, y=w4674) -> (x/y=w4675:dbl[])
            n2699 = Divide(x=w4673, y=w4671) -> (x/y=w4672:dbl[])
            n2700 = Build Array(w4688, w4687, w4702, w4686, w4685, w4699, w4675, w4674, w4672, w4671, w4668, w4667, w4666) -> (w4665:dbl[][])
            n2701 = Bundle("T1 Y", "T1 X", "T1 Sum", "T2 Y", "T2 X", "T2 Sum", "T1 FB X", "T1 FB Sum", "T2 FB X", "T2 FB Sum", "PSD Y", "PSD X", "PSD Y Sum") -> (w4689:T49)  [unwired: 1 out]
            n2702 = Cluster To Array(cluster=w4689) -> (array=w4698:string[])
          }
          frame "IR-QPD + PSD + FB-QPD XY positions" {
            w4763 = 4  # Channel pattern
            # "time average x2 the 3 psd signals (detection laser)"
            # "deinterlace 3 signals from qpds"
            n2703 = Decimate 1D Array(w4779) -> (w4778:i16[], w4777:i16[], w4764:i16[], w4776:i16[], w4734:i16[], w4752:i16[])  [unwired: 2 out]
            n2704 = Decimate 1D Array "Feedback Sum"(w4764) -> (w4715:i16[], w4712:i16[])
            n2705 = Decimate 1D Array "QPD Y"(w4778) -> (w4723:i16[], w4720:i16[])
            n2706 = Decimate 1D Array "QPD X"(w4777) -> (w4722:i16[], w4719:i16[])
            n2707 = Decimate 1D Array "Feedback Y"(w4734) -> (w4717:i16[], w4714:i16[])
            n2708 = Decimate 1D Array "QPD Sum"(w4776) -> (w4721:i16[], w4718:i16[])
            n2709 = Decimate 1D Array "Feedback X"(w4752) -> (w4716:i16[], w4713:i16[])
            n2710 = call "downsample 1D array - double.vi"("Ave N"=2.0) -> ("Array Out"=w4751:dbl[])  [unwired: 1 in, 1 out]
            n2711 = call "downsample 1D array - double.vi"("Ave N"=2.0) -> ("Array Out"=w4750:dbl[])  [unwired: 1 in, 1 out]
            n2712 = Interleave 1D Arrays(w4723, w4722, w4721, w4720, w4719, w4718, w4717, w4716, w4715, w4714, w4713, w4712, w4751, w4750) -> (w4773:dbl[])
            n2713 = Divide(x=w4773, y=3276.7) -> (x/y=w4772:dbl[])
            n2714 = Decimate 1D Array(w4772) -> (w4771:dbl[], w4770:dbl[], w4769:dbl[], w4768:dbl[], w4767:dbl[], w4766:dbl[], w4731:dbl[], w4743:dbl[], w4729:dbl[], w4730:dbl[], w4741:dbl[], w4727:dbl[], w4739:dbl[], w4737:dbl[])
            n2715 = Negate(x=w4737) -> (-x=w4735:dbl[])
            n2716 = Divide(x=w4739, y=w4735) -> (x/y=w4738:dbl[])
            n2717 = Divide(x=w4730, y=w4727) -> (x/y=w4726:dbl[])
            n2718 = Divide(x=w4731, y=w4729) -> (x/y=w4728:dbl[])
            n2719 = Divide(x=w4771, y=w4769) -> (x/y=w4756:dbl[])
            n2720 = Divide(x=w4770, y=w4769) -> (x/y=w4755:dbl[])
            n2721 = Divide(x=w4768, y=w4766) -> (x/y=w4754:dbl[])
            n2722 = Divide(x=w4767, y=w4766) -> (x/y=w4753:dbl[])
            n2723 = Divide(x=w4743, y=w4729) -> (x/y=w4742:dbl[])
            n2724 = Divide(x=w4741, y=w4727) -> (x/y=w4740:dbl[])
            n2725 = Build Array(w4756, w4755, w4769, w4754, w4753, w4766, w4728, w4742, w4729, w4726, w4740, w4727, w4738, w4737) -> (w4736:dbl[][])
            n2726 = Bundle("T1 Y", "T1 X", "T1 Sum", "T2 Y", "T2 X", "T2 Sum", "T1 FB Y", "T1 FB X", "T1 FB Sum", "T2 FB Y", "T2 FB X", "T2 FB Sum", "PSD X", "PSD Y Sum") -> (w4725:T50)  [unwired: 1 out]
            n2727 = To Word Integer(number=w4773) -> (16bit integer=w4724:i16[])
            n2728 = Cluster To Array(cluster=w4725) -> (array=w4765:string[])
          }
        }
      }
    }
    "AI labels" <- w3796
    n2729 = Decimate 1D Array(w3774) -> (w3584:u32[], w3585:u32[])
    n2730 = local read "DMA Update Period (s)"() -> (w3805:dbl)
    n2731 = Build Array(w3584, w3585) -> (w3588:u32[][])
    n2732 = local read "Data Period (s)"() -> (w3659:dbl)
    n2733 = local read "BD 1 Frequency 2 (MHz)"() -> (w3692:dbl)
    n2734 = local read "BD 1 Frequency 1 (MHz)"() -> (w3693:dbl)
    n2735 = Decimate 1D Array(w3700) -> (w3720:i16[], w3719:i16[], w3717:i16[], w3716:i16[])  [unwired: 9 out]
    n2736 = To Double Precision Float(number=w3588) -> (double precision float=w3862:dbl[][])
    n2737 = local read "APD Integration Time (s)"() -> (w3756:dbl)
    n2738 = Multiply(x=w3659, y="Trap Pos. Disp. Downsample") -> (x*y=w3657:dbl)
    n2739 = Divide(x=w3720, y=w3719) -> (x/y=w3721:dbl[])
    n2740 = Divide(x=w3717, y=w3716) -> (x/y=w3718:dbl[])
    n2741 = feedback #10(0.0) -> (w3734:dbl)
    n2742 = Add(x=w3805, y=w3734) -> (x+y=w3899:dbl)
    n2743 = feedback-in #10(w3899) -> ()
    n2744 = local read "AOM X Cal (nm/MHz)"() -> (w3690:dbl)
    n2745 = To Time Stamp(1:w3734) -> (0:w3733:timestamp)
    n2746 = Split 1D Array(array=w3721, index="N El. to Ave.") -> (second subarray=w3724:dbl[])  [unwired: 1 out]
    n2747 = Split 1D Array(array=w3718, index="N El. to Ave.") -> (second subarray=w3723:dbl[])  [unwired: 1 out]
    n2748 = Multiply(x=w3659, y="Trap Disp. Downsample") -> (x*y=w3735:dbl)
    "Display Period (s)" <- w3735
    n2749 = for "Trap AI" {
      tunnel: [w4511] -> w3893 mode=indexing
      tunnel: w3733 -> [w4501]
      tunnel: "Trap Disp. Downsample" -> [w4509]
      tunnel: w3797 -> [w4507] mode=indexing
      tunnel: w3659 -> [w4506]
      tunnel: w3796 -> [w4505] mode=indexing
      tunnel: w3732 -> [w4504]
      tunnel: [w4503] -> w3766 mode=indexing
      tunnel: w3735 -> [w4502]
      workers-P: _ -> [_]
      n2750 = Bundle By Name("Y"=w4507, "dt"=w4506) -> (w4508:waveform(dbl))  [unwired: 1 out]
      n2751 = Set Waveform Attribute(5:w4505, 6:w4504, 7:w4508) -> (3:w4503:waveform(dbl))  [unwired: 1 in, 2 out]
      n2752 = call "downsample 1D array - double.vi"("Ave N"=w4509, "Array In"=w4507) -> ("Array Out"=w4510:dbl[])  [unwired: 1 out]
      n2753 = Bundle By Name(cluster=w4503, "t0"=w4501, "Y"=w4510, "dt"=w4502) -> (w4511:waveform(dbl))
    }
    n2754 = Bundle("BD 1 Frequency 1 (MHz)"=w3693, "BD 1 Frequency 2 (MHz)"=w3692) -> (w3694:T51)  [unwired: 1 out]
    n2755 = call-poly <vilib>:"Mean.vi"("X"=w3723) -> ("mean"=w3711:dbl)  [unwired: 1 out]
    n2756 = call-poly <vilib>:"Mean.vi"("X"=w3724) -> ("mean"=w3712:dbl)  [unwired: 1 out]
    n2757 = Reciprocal(x=w3735) -> (1/x=→"Trap Disp. Freq. (Hz)":dbl)
    n2758 = Cluster To Array(cluster=w3694) -> (array=w3691:dbl[])
    n2759 = local read "Trap X AI1 (DMA)"() -> (w3722:T13)
    n2760 = local read "Data points/scans (MCL)"() -> (w3873:dbl)
    n2761 = To Fixed-Point(number=w3711) -> (fixed-point=w3709:fxp<+/-,16,1>)  [unwired: 1 in]
    n2762 = To Fixed-Point(number=w3712) -> (fixed-point=w3710:fxp<+/-,16,1>)  [unwired: 1 in]
    n2763 = Bundle("Trap 1 Pos.", "Trap 2 Pos.") -> (w3731:cluster{string, string})  [unwired: 1 out]
    n2764 = Bundle By Name(cluster=w3722, "Set 1"=w3710, "Set 2"=w3709) -> (→"Trap X AI1 (DMA)":T13)
    n2765 = Cluster To Array(cluster=w3731) -> (array=w3728:string[])
    n2766 = Bundle("APD 1", "APD 2") -> (w3892:cluster{string, string})  [unwired: 1 out]
    n2767 = Select(t=-1.0, s="Negate Y Axis", f=1.0) -> (s? t:f=w3676:dbl)
    n2768 = for "Trap Position" {
      tunnel: w3737 -> [w4143] mode=indexing
      tunnel: "Trap Pos. Disp. Downsample" -> [w4142]
      tunnel: w3657 -> [w4140]
      tunnel: w3733 -> [w4139]
      tunnel: w3732 -> [w4137]
      tunnel: w3728 -> [w4136] mode=indexing
      tunnel: [w4135] -> w3646 mode=indexing
      tunnel: w3691 -> [w4133] mode=indexing
      tunnel: w3690 -> [w4131]
      tunnel: w3676 -> [w4130]
      n2769 = call "downsample 1D array - double.vi"("Ave N"=w4142, "Array In"=w4143) -> ("Array Out"=w4141:dbl[])  [unwired: 1 out]
      n2770 = Subtract(x=w4141, y=w4133) -> (x-y=w4134:dbl[])
      n2771 = Multiply(x=w4131, y=w4134) -> (x*y=w4132:dbl[])
      n2772 = Multiply(x=w4130, y=w4132) -> (x*y=w4129:dbl[])
      n2773 = Bundle By Name("Y"=w4129, "dt"=w4140, "t0"=w4139) -> (w4138:waveform(dbl))  [unwired: 1 out]
      n2774 = Set Waveform Attribute(5:w4136, 6:w4137, 7:w4138) -> (3:w4135:waveform(dbl))  [unwired: 1 in, 2 out]
    }
    n2775 = Cluster To Array(cluster=w3892) -> (array=w3889:string[])
    n2776 = for "APD" {
      tunnel: w3862 -> [w4487] mode=indexing
      tunnel: w3756 -> [w4498]
      tunnel: [w4494] -> w3762 mode=indexing
      tunnel: "APD Disp. Scale" -> [w4495]
      tunnel: w3732 -> [w4493]
      tunnel: w3889 -> [w4492] mode=indexing
      tunnel: "APD Disp. Downsample" -> [w4489]
      tunnel: [w4491] -> w3888
      workers-P: _ -> [_]
      tunnel: w3733 -> [w4488]
      n2777 = call "integrate 1D array interval - double.vi"("Ave N"=w4489, "Array In"=w4487) -> ("Array Out"=w4490:dbl[])  [unwired: 1 out]
      n2778 = Multiply(x=w4498, y=w4489) -> (x*y=w4491:dbl)
      n2779 = Divide(x=w4490, y=w4495) -> (x/y=w4496:dbl[])
      n2780 = Bundle By Name("t0"=w4488, "Y"=w4496, "dt"=w4491) -> (w4497:waveform(dbl))  [unwired: 1 out]
      n2781 = Set Waveform Attribute(5:w4492, 6:w4493, 7:w4497) -> (3:w4494:waveform(dbl))  [unwired: 1 in, 2 out]
    }
    "APD Display Period (s)" <- w3888
    n2782 = Reciprocal(x=w3888) -> (1/x=→"APD Display Freq. (Hz)":dbl)
    n2783 = local read "Display Period (s)"() -> (w3783:dbl)
    n2784 = Increment(x=w3873) -> (x+1=w3874:dbl)
    n2785 = To Double Precision Float(number=w3584) -> (double precision float=w3794:dbl[])
    n2786 = Index Array(array=w3646, index=0) -> (element=w3650:waveform(dbl))
    n2787 = Index Array(array=w3646, index=1) -> (element=w3645:waveform(dbl))
    n2788 = feedback #11(w3874) -> (w3877:dbl)
    n2789 = Select(t=0, s=w3864, f=w3877) -> (s? t:f=w3870:dbl)
    n2790 = Array Size(array=w3794) -> (size(s)=w3876:i32)
    n2791 = Add(x=w3876, y=w3870) -> (x+y=w3871:dbl)
    n2792 = Unbundle By Name(w3650) -> ("Y"=w3651:dbl[])
    n2793 = feedback #12(w3584) -> (w3861:u32[])
    n2794 = Build Array (concatenate)(w3861, w3584) -> (w3858:u32[])
    n2795 = feedback #13(w3585) -> (w3761:u32[])
    n2796 = Divide(x="Bead Sep. Int. Time (s)", y=w3783) -> (x/y=w3686:dbl)
    n2797 = Build Array (concatenate)(w3761, w3585) -> (w3760:u32[])
    n2798 = Add(x=w3651, y="FB Trap Pos Offset") -> (x+y=w3649:dbl[])
    "T1 x pos data" <- w3649
    n2799 = Greater?(x=w3871, y=w3873) -> (0:w3872:bool)
    n2800 = feedback #14(w3649) -> (w3688:dbl[])
    n2801 = Build Array (concatenate)(w3649, w3688) -> (w3687:dbl[])
    n2802 = Bundle By Name(cluster=w3650, "Y"=w3649) -> (w3648:waveform(dbl))
    n2803 = Select(t=w3870, s=w3872, f=w3871) -> (s? t:f=w3869:dbl)
    n2804 = feedback-in #11(w3869) -> ()
    n2805 = Array Size(array=w3858) -> (size(s)=w3855:i32)
    n2806 = Array Size(array=w3584) -> (size(s)=w3857:i32)
    n2807 = local read "MCL Scanning"() -> (w3867:bool)
    n2808 = local read "APD Integration Time (s)"() -> (w3769:dbl)
    n2809 = Bundle(w3648, w3645) -> (w3644:cluster{waveform(dbl), waveform(dbl)})  [unwired: 1 out]
    n2810 = Build Array (concatenate)(w3762, w3893) -> (w3764:waveform(dbl)[])
    "All Signals" <- w3764
    n2811 = Split 1D Array(array=w3687, index=w3686) -> (first subarray=w3680:dbl[])  [unwired: 1 out]
    n2812 = feedback-in #14(w3680) -> ()
    n2813 = Multiply(x=w3857, y="APD Ave N") -> (x*y=w3856:dbl)
    n2814 = Greater?(x=w3855, y=w3856) -> (0:w3859:bool)
    n2815 = Not(x=w3872) -> (.not. x?=w3866:bool)
    n2816 = Cluster To Array(cluster=w3644) -> (array=w3620:waveform(dbl)[])
    "Trap Positions" <- w3620
    n2817 = To Double Precision Float(number=w3585) -> (double precision float=w3743:dbl[])
    n2818 = call-poly <vilib>:"Mean.vi"("X"=w3680) -> ("mean"=w3679:dbl)  [unwired: 1 out]
    "Mean T1 Position (nm)" <- w3679
    n2819 = Subtract(x=w3680, y=w3679) -> (x-y=w3685:dbl[])
    n2820 = Square(x=w3685) -> (x^2=w3684:dbl[])
    n2821 = And(x=w3866, y=w3867) -> (x .and. y?=w3868:bool)
    n2822 = call-poly <vilib>:"Mean.vi"("X"=w3684) -> ("mean"=w3683:dbl)  [unwired: 1 out]
    n2823 = case shown="True" w3859 {
      tunnel: w3858 -> [w4270 w4272]
      tunnel: [w4270 w4276] -> w3586
      tunnel: w3856 -> [_ w4274]
      tunnel: w3855 -> [_ w4277]
      tunnel: w3760 -> [w4269 w4271]
      tunnel: [w4269 w4273] -> w3587
      frame False {
      }
      frame True {
        n2824 = Subtract(x=w4277, y=w4274) -> (x-y=w4275:dbl)
        n2825 = Array Subset(array=w4272, index=w4275, length=w4274) -> (w4276:u32[])
        n2826 = Array Subset(array=w4271, index=w4275, length=w4274) -> (w4273:u32[])
      }
